vi "浊度电极校准.vi"() -> ()   [LabVIEW 2016, in "斯坦道多参数.lvlib"]
uses:
  <vilib>/Utility/miscctls.llb/LVPointTypeDef.ctl
  <vilib>/Utility/miscctls.llb/LVPositionTypeDef.ctl
  <vilib>/Analysis/NI_AALBase.lvlib
panel:
  out "第三点校准值":dbl
  out "标液3":dbl
  out "第二点校准值":dbl
  out "第一点校准值":dbl
  in  "校准停止":bool
  in  "校准启动":bool
  in  "校准模式":enum16{"两点校准", "单点校准", "三点校准"}(ring)
  out "最小值":sgl format="%#.2f"
  out "最大值":sgl format="%#.2f"
  out "波形图表":sgl(graph) caption="历史曲线"
  out "mean":dbl caption="均值" format="%#.2f"
  out "standard deviation":dbl caption="标准差" format="%#.2f"
  out "变异系数":dbl format="%#.6f"
  out "测量值":dbl
  out "提示":string
  out "标液2":dbl
  out "标液1":dbl
  out "原始读取值":dbl caption="信号值"
  out "偏移值补偿":dbl
  out "电极斜率":dbl
  out "电极零点":dbl
  # "浊度电极设定"
  # "NTU"
  # "%"
  # "NTU"
  # "NTU"
  # "NTU"
  # "请选择校准模式:"
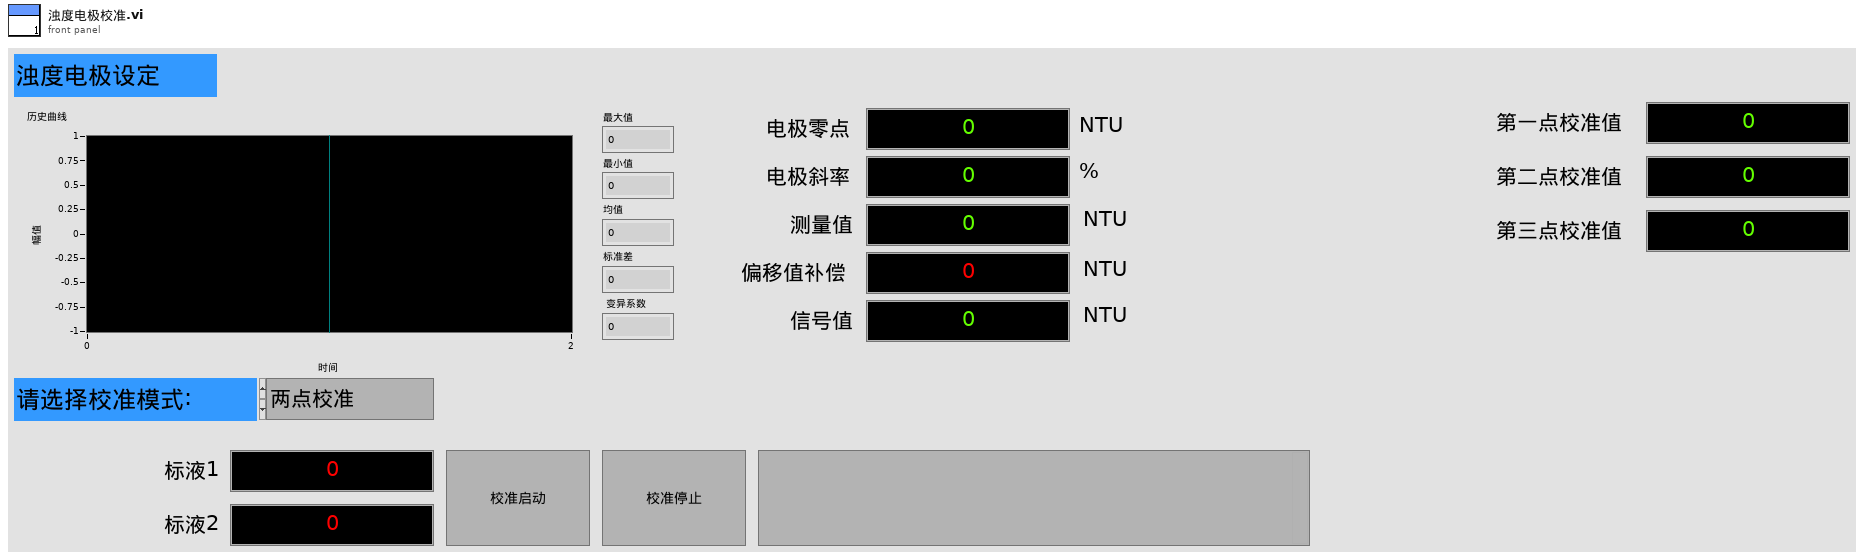
[diagram p1: front panel]
types:
  T1 = typedef "LVPointTypeDef.ctl" = cluster{"Horizontal":i16, "Vertical":i16}
  T2 = typedef "斯坦道多参数.lvlib/校准步骤.ctl" = enum16{"待机", "放置第一点标液", "第一点校准启动", "第一点校准写入", "第一点校准失败", "放置第二点标液", "第二点校准启动", "第二点校准写入", "第二点校准失败", "放置第三点标液", "第三点校准启动", "第三点校准写入", "第三点校准失败", "校准结果写入", "校准结束"}
  T3 = cluster{"电极状态标志":u16, "电极型号标志":u16, "浊度测量值":sgl, "温度测量值":sgl, "浊度信号值":sgl, "浊度偏移修正值":sgl, "温度偏移修正值":sgl, "手动温度补偿值":sgl, "浊度电极零点":sgl, "浊度电极斜率":sgl, "第1点标准值记录":sgl, "第1点信号值记录":sgl, "第1点温度值记录":sgl, "第2点标准值记录":sgl, "第2点信号值记录":sgl, "第2点温度值记录":sgl, "命令滤波设定":u16, "温度模式":enum16{"ATC", "MTC"}, "生产批次":u16, "电极序号":u16, "串口地址":u16, "串口波特率":enum16{"9600", "19200", "115200"}, "串口校验位":enum16{"NONE", "ODD", "EVEN"}, "串口停止位":enum16{"1bit", "2bit"}, "第一点标准值":sgl, "第二点标准值":sgl, "第三点标准值":sgl}
  T4 = typedef "LVPositionTypeDef.ctl" = cluster{"Left":i32, "Top":i32}
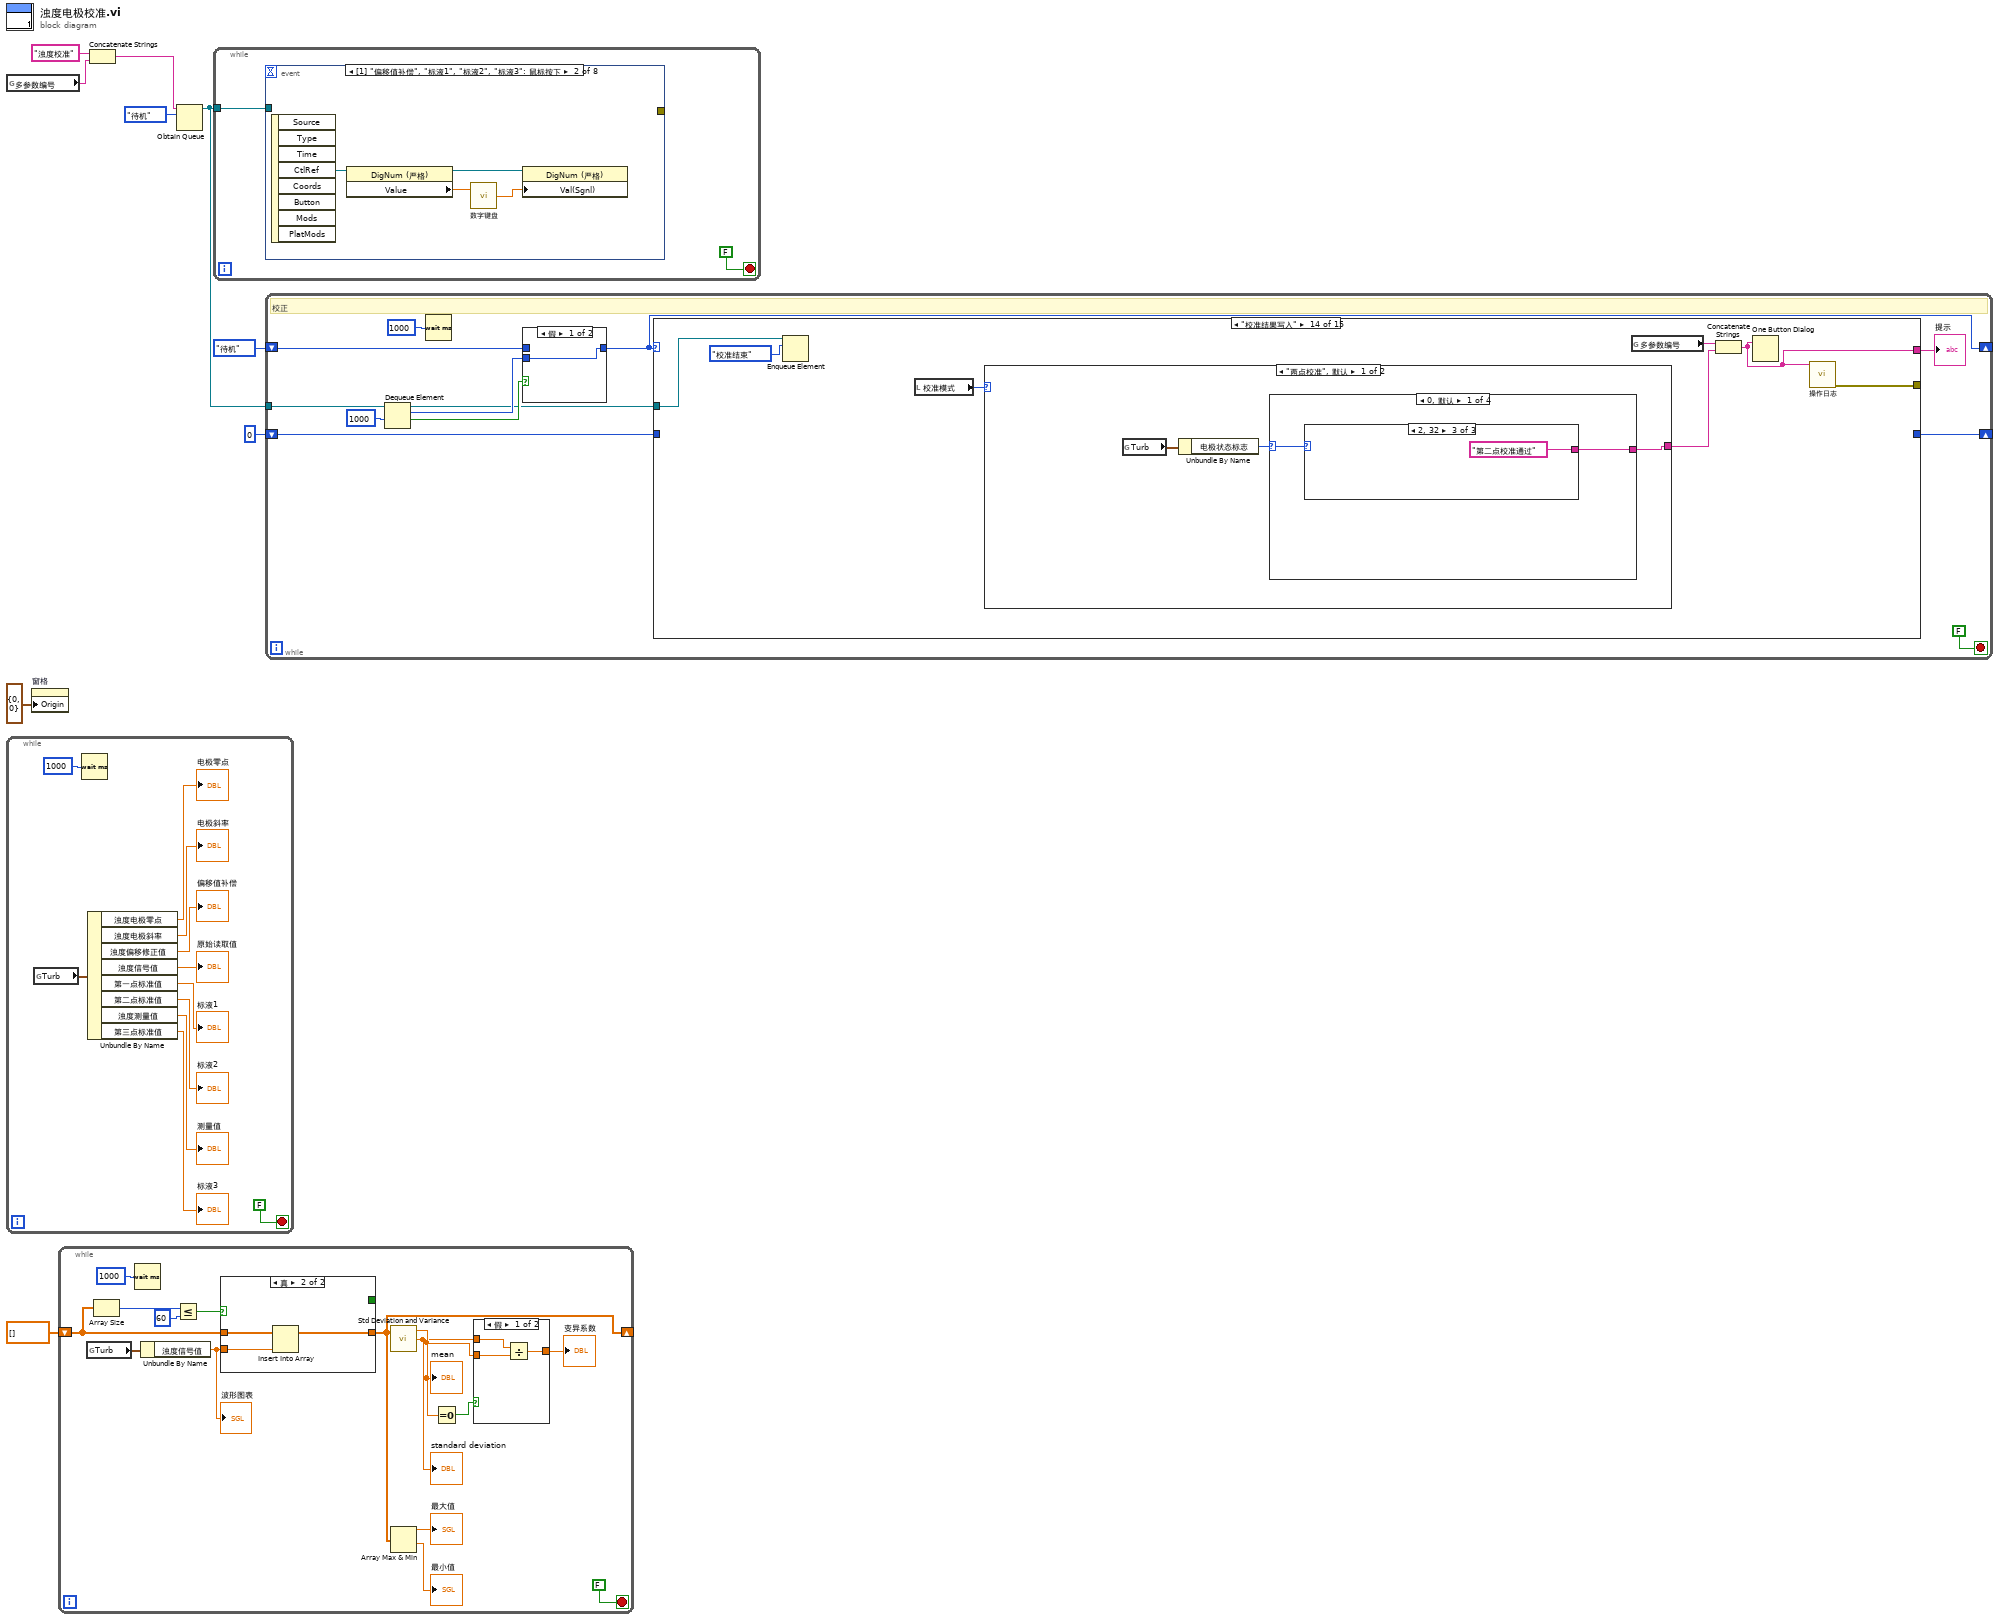
[diagram p0: block diagram]
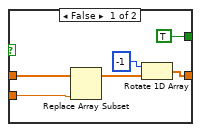
[diagram p3: hidden frame]
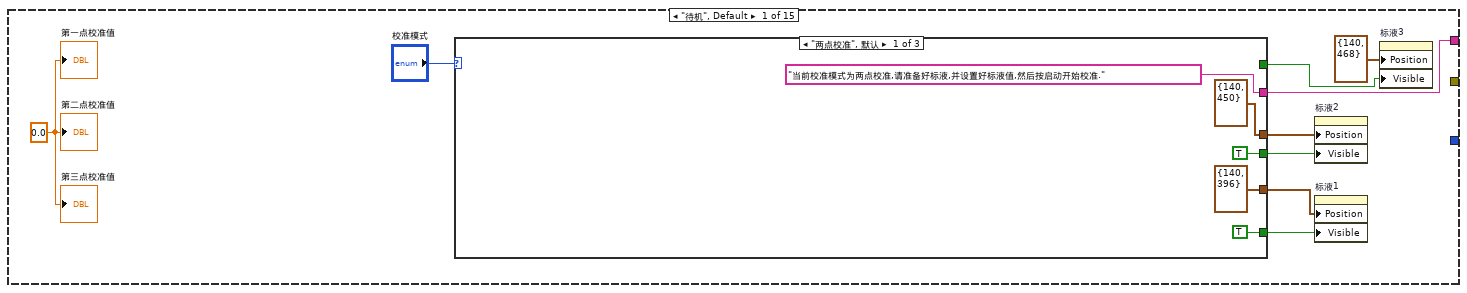
[diagram p5: hidden frame]
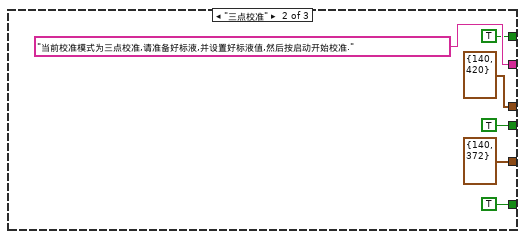
[diagram p6: hidden frame]
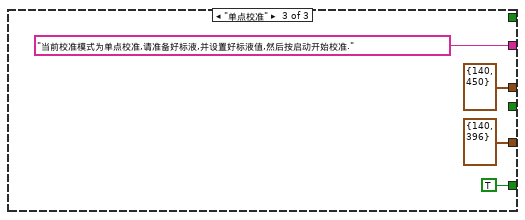
[diagram p7: hidden frame]
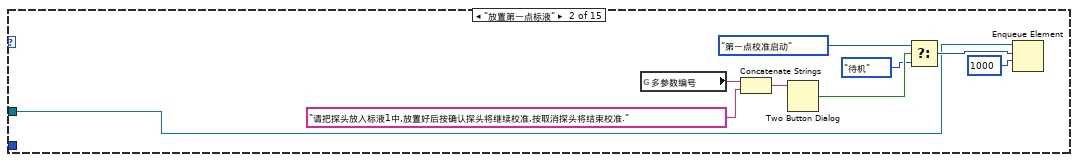
[diagram p8: hidden frame]
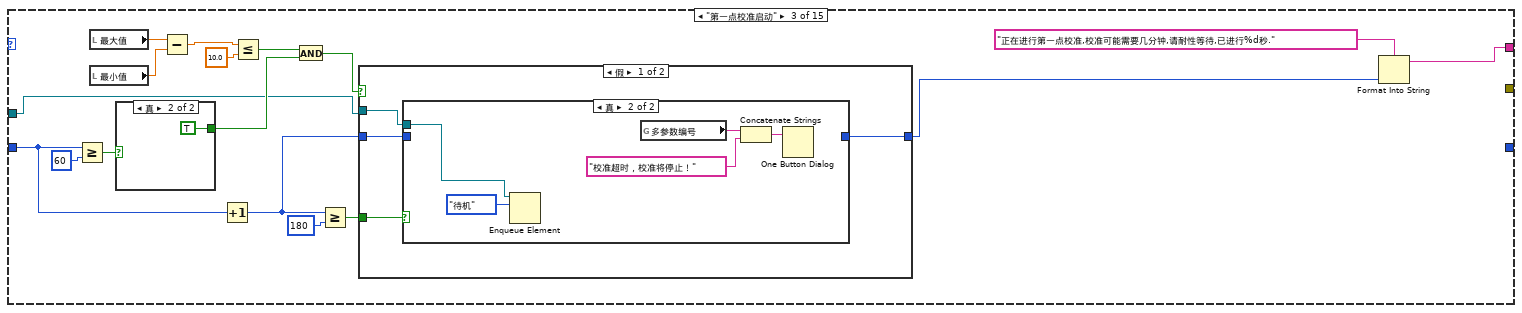
[diagram p9: hidden frame]
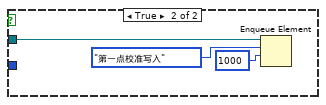
[diagram p11: hidden frame]
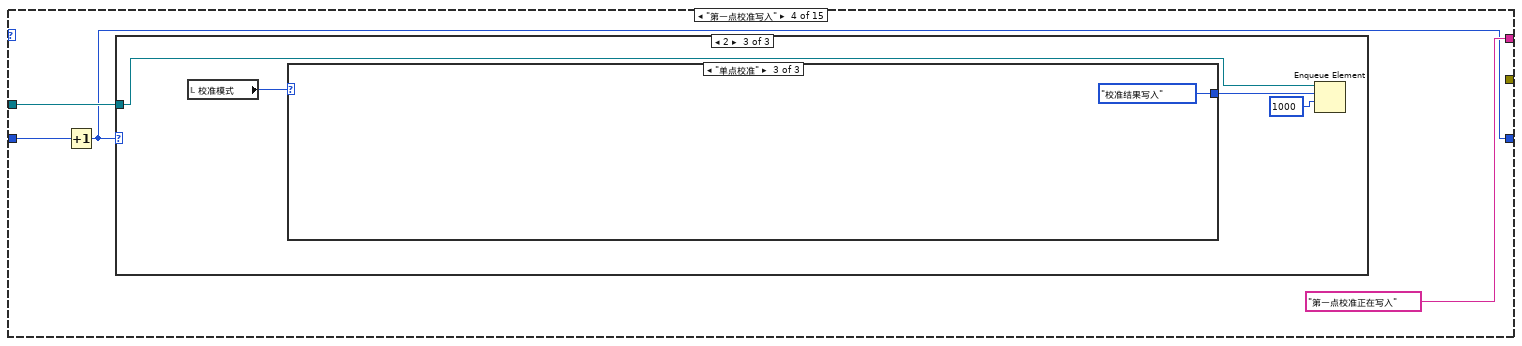
[diagram p13: hidden frame]
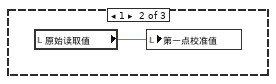
[diagram p15: hidden frame]
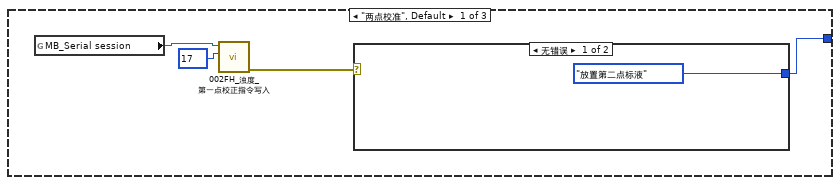
[diagram p16: hidden frame]
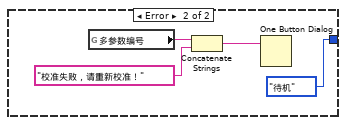
[diagram p17: hidden frame]
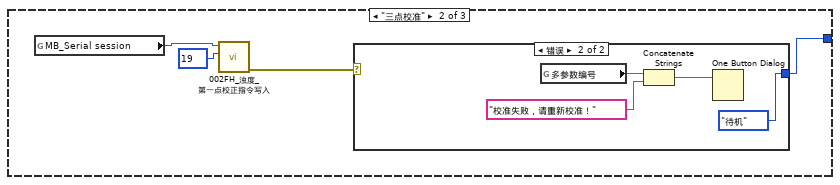
[diagram p18: hidden frame]
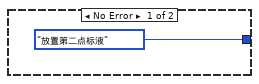
[diagram p19: hidden frame]
diagram:
  n1 = global read "多参数全局变量.vi" "多参数编号"() -> (w1:string)
  n2 = while {
    stop <- FALSE stop-if-true
    n3 = global read "国弘过程全局变量.vi" "Turb"() -> (w18:T3)
    n4 = Wait (ms)(milliseconds to wait=u32 1000 ("等待时间（毫秒）")) -> ()  [unwired: 1 out]
    n5 = Unbundle By Name(w18) -> ("浊度电极零点"=→"电极零点":sgl, "浊度电极斜率"=→"电极斜率":sgl, "浊度偏移修正值"=→"偏移值补偿":sgl, "浊度信号值"=→"原始读取值":sgl, "第一点标准值"=→"标液1":sgl, "第二点标准值"=→"标液2":sgl, "浊度测量值"=→"测量值":sgl, "第三点标准值"=→"标液3":sgl)
  }
  n6 = property on="窗格" class="Pane"("Origin"=T1 {"Horizontal"=0, "Vertical"=0} ("原点")) -> ()  [unwired: 2 in, 2 out]
  n7 = while {
    shift-right: [w24] -> _
    shift-left: sgl[] [] -> [w31]
    stop <- FALSE stop-if-true
    n8 = global read "国弘过程全局变量.vi" "Turb"() -> (w25:T3)
    n9 = Array Size(array=w31) -> (size(s)=w33:i32)
    n10 = Wait (ms)(milliseconds to wait=u32 1000 ("等待时间（毫秒）")) -> ()  [unwired: 1 out]
    n11 = Unbundle By Name(w25) -> ("浊度信号值"=w21:sgl)
    "波形图表" <- w21
    n12 = Less Or Equal?(x=w33, y=60) -> (x <= y?=w32:bool)
    n13 = case shown="真" w32 {
      tunnel: w31 -> [w44 w47]
      tunnel: w21 -> [w42 w46]
      tunnel: [w40 w45] -> w24
      tunnel: [TRUE _] -> _
      frame False {
        n14 = Replace Array Subset(array=w44, new element=w42) -> (w43:sgl[])  [unwired: 1 in]
        n15 = Rotate 1D Array(1:w43, 2:-1 ("n")) -> (0:w40:sgl[])
      }
      frame True {
        n16 = Insert Into Array(array=w47, new element=w46) -> (w45:sgl[])  [unwired: 1 in]
      }
    }
    n17 = call <vilib>:"Std Deviation and Variance.vi"("X"=w24) -> ("mean"=w29:dbl, "standard deviation"=w28:dbl)  [unwired: 1 in, 1 out]
    "mean" <- w29
    "standard deviation" <- w28
    n18 = Array Max & Min(array=w24) -> (max value=→"最大值":sgl, min value=→"最小值":sgl)  [unwired: 2 out]
    n19 = Equal To 0?(x=w29) -> (x = 0?=w30:bool)
    n20 = case shown="假" w30 {
      tunnel: w28 -> [w38 _]
      tunnel: [w37 _] -> w27
      tunnel: w29 -> [w36 _]
      frame False {
        n21 = Divide(x=w38, y=w36) -> (x/y=w37:dbl)
      }
      frame True {
      }
    }
    "变异系数" <- w27
  }
  n22 = Concatenate Strings("浊度校准" ("名称（未命名）"), w1) -> (w2:string)
  n23 = Obtain Queue(name (unnamed)=w2, element data type=校准步骤."待机" ("枚举")) -> (queue out=w4:refnum<queue>)  [unwired: 3 in, 2 out]
  n24 = while {
    tunnel: w4 -> [w48]
    stop <- FALSE stop-if-true
    n25 = event shown="[1] \"偏移值补偿\", \"标液1\", \"标液2\", \"标液3\": 鼠标按下" {
      selector: _ -> [_ _ _ _ _ _ _ _]
      dyn-events: _ -> [_ _ _ _ _ _ _ _]
      timeout: _ -> [_ _ _ _ _ _ _ _]
      tunnel: [_ _ w55 w58 w62 w65 _ _] -> _
      tunnel: w48 -> [_ _ _ _ _ _ w66 w68]
      event Timeout {
        n26 = event-data() -> ()  [unwired: 1 in, 3 out]
      }
      event "偏移值补偿", "标液1", "标液2", "标液3": Mouse Down {
        n27 = event-data() -> ("CtlRef"=w50:refnum<vi>)  [unwired: 1 in, 7 out]
        n28 = property class="DigNum (严格)"(reference=w50) -> (reference out=w51:refnum<vi>, "Value"=w52:dbl)  [unwired: 1 in, 1 out]
        n29 = call "数字键盘.vi"("OldNumber"=w52) -> ("NewNumber"=w53:dbl)  [unwired: 1 in]
        n30 = property class="DigNum (严格)"(reference=w51, "Val(Sgnl)"=w53) -> ()  [unwired: 1 in, 2 out]
      }
      event "偏移值补偿": Value Change {
        n31 = event-data() -> ("NewVal"=w56:dbl)  [unwired: 1 in, 5 out]
        n32 = global read "多参数全局变量.vi" "MB_Serial session"() -> (w54:refnum<class "MB_Master_Serial.lvclass">)
        n33 = call "000CH_浊度_浊度偏移修正值写入.vi"("数值"=w56, "MB_Serial session in"=w54) -> ("error out"=w55:errorcluster)  [unwired: 8 in, 1 out]
      }
      event "标液1": Value Change {
        n34 = event-data() -> ("NewVal"=w59:dbl)  [unwired: 1 in, 5 out]
        n35 = global read "多参数全局变量.vi" "MB_Serial session"() -> (w57:refnum<class "MB_Master_Serial.lvclass">)
        n36 = call "0030H_浊度_第一点标准值写入.vi"("数值"=w59, "MB_Serial session in"=w57) -> ("error out"=w58:errorcluster)  [unwired: 8 in, 1 out]
      }
      event "标液2": Value Change {
        n37 = event-data() -> ("NewVal"=w61:dbl)  [unwired: 1 in, 5 out]
        n38 = global read "多参数全局变量.vi" "MB_Serial session"() -> (w60:refnum<class "MB_Master_Serial.lvclass">)
        n39 = call "0033H_浊度_第二点标准值写入.vi"("数值"=w61, "MB_Serial session in"=w60) -> ("error out"=w62:errorcluster)  [unwired: 8 in, 1 out]
      }
      event "标液3": Value Change {
        n40 = event-data() -> ("NewVal"=w64:dbl)  [unwired: 1 in, 5 out]
        n41 = global read "多参数全局变量.vi" "MB_Serial session"() -> (w63:refnum<class "MB_Master_Serial.lvclass">)
        n42 = call "0036H_浊度_第三点标准值写入.vi"("数值"=w64, "MB_Serial session in"=w63) -> ("error out"=w65:errorcluster)  [unwired: 8 in, 1 out]
      }
      event "校准启动": Value Change {
        n43 = event-data() -> ()  [unwired: 1 in, 6 out]
        n44 = Enqueue Element(queue=w66, element=校准步骤."放置第一点标液" ("元素")) -> ()  [unwired: 2 in, 3 out]
      }
      event "校准停止": Value Change {
        n45 = event-data() -> ()  [unwired: 1 in, 6 out]
        n46 = Flush Queue(queue=w68) -> (queue out=w69:refnum<queue>)  [unwired: 1 in, 2 out]
        n47 = Enqueue Element(queue=w69, element=校准步骤."待机" ("元素"), timeout in ms (-1)=1000 ("超时毫秒(-1)")) -> ()  [unwired: 1 in, 3 out]
      }
    }
  }
  n48 = while "While循环" {
    shift-right: [w73] -> _
    shift-left: 校准步骤."待机" ("枚举") -> [w75]
    shift-right: [w72] -> _
    shift-left: 0 -> [w81]
    tunnel: w4 -> [w76]
    stop <- FALSE stop-if-true
    # "校正"
    n49 = Dequeue Element(queue=w76, timeout in ms (-1)=1000 ("超时毫秒(-1)")) -> (queue out=w74:refnum<queue>, element=w77:T2, timed out?=w78:bool)  [unwired: 1 in, 1 out]
    n50 = Wait (ms)(milliseconds to wait=u32 1000 ("等待时间（毫秒）")) -> ()  [unwired: 1 out]
    n51 = case shown="假" w78 {
      tunnel: w77 -> [w84 _]
      tunnel: [w84 w85] -> w73
      tunnel: w75 -> [_ w85]
      frame False {
      }
      frame True {
      }
    }
    n52 = case shown="\"校准结果写入\"" w73 {
      tunnel: [w93 _ w119 "第一点校准正在写入" ("提示") _ _ w189 "第二点校准正在写入" ("提示") "第二点校准失败" ("提示") _ "第三点校准正在写入" ("提示") w273 "第三点校准失败" ("提示") w304 w342] -> w80
      tunnel: w81 -> [_ _ w121 w152 _ _ w190 w220 _ _ w257 w274 _ _ _]
      tunnel: [_ _ _ w150 _ _ w188 w218 _ _ w255 w272 _ _ _] -> w72
      tunnel: w74 -> [_ w112 w122 w151 _ w180 w191 w219 _ w248 w256 w275 _ w308 _]
      tunnel: [_ _ _ _ _ _ _ _ _ _ _ _ _ w303 _] -> _
      frame "待机", Default {
        w86 = 0.0 ("第一点校准值")
        n53 = case shown="\"两点校准\", 默认" "校准模式" {
          tunnel: ["当前校准模式为两点校准,请准备好标液,并设置好标液值,然后按启动开始校准." ("提示") "当前校准模式为三点校准,请准备好标液,并设置好标液值,然后按启动开始校准." ("提示") "当前校准模式为单点校准,请准备好标液,并设置好标液值,然后按启动开始校准." ("提示")] -> w93
          tunnel: [TRUE ("可见") TRUE ("可见") _] -> w89
          tunnel: [T4 {"Left"=140, "Top"=396} ("位置") T4 {"Left"=140, "Top"=372} ("位置") T4 {"Left"=140, "Top"=396} ("位置")] -> w92
          tunnel: [T4 {"Left"=140, "Top"=450} ("位置 2") T4 {"Left"=140, "Top"=420} ("位置 2") T4 {"Left"=140, "Top"=450} ("位置 2")] -> w91
          tunnel: [_ TRUE ("可见") _] -> w88
          tunnel: [TRUE ("可见") TRUE ("可见") TRUE ("可见")] -> w87
          frame "两点校准", Default {
          }
          frame "三点校准" {
          }
          frame "单点校准" {
          }
        }
        n54 = property on="标液2" class="DigNum (严格)"("Position"=w91, "Visible"=w89) -> ()  [unwired: 2 in, 2 out]
        n55 = property on="标液1" class="DigNum (严格)"("Position"=w92, "Visible"=w87) -> ()  [unwired: 2 in, 2 out]
        n56 = property on="标液3" class="DigNum (严格)"("Position"=T4 {"Left"=140, "Top"=468} ("位置 3"), "Visible"=w88) -> ()  [unwired: 2 in, 2 out]
        "第一点校准值" <- w86
        "第二点校准值" <- w86
        "第三点校准值" <- w86
      }
      frame "放置第一点标液" {
        n57 = global read "多参数全局变量.vi" "多参数编号"() -> (w110:string)
        n58 = Concatenate Strings(w110, "请把探头放入标液1中,放置好后按确认探头将继续校准,按取消探头将结束校准." ("消息")) -> (w111:string)
        n59 = Two Button Dialog(message=w111) -> (T button?=w116:bool)  [unwired: 2 in]
        n60 = Select(t=校准步骤."第一点校准启动" ("元素"), s=w116, f=校准步骤."待机" ("元素")) -> (s? t:f=w113:T2)
        n61 = Enqueue Element(queue=w112, element=w113, timeout in ms (-1)=1000 ("超时毫秒(-1)")) -> ()  [unwired: 1 in, 3 out]
      }
      frame "第一点校准启动" {
        n62 = Greater Or Equal?(x=w121, y=60) -> (x >= y?=w128:bool)
        n63 = local read "最大值"() -> (w131:sgl)
        n64 = local read "最小值"() -> (w130:sgl)
        n65 = case shown="真" w128 {
          tunnel: [_ TRUE] -> w129
          frame False {
          }
          frame True {
          }
        }
        n66 = Subtract(x=w131, y=w130) -> (x-y=w132:sgl)
        n67 = Increment(x=w121) -> (x+1=w135:i32)
        n68 = Less Or Equal?(x=w132, y=10.0) -> (x <= y?=w125:bool)
        n69 = And(x=w125, y=w129) -> (x .and. y?=w133:bool)
        n70 = Greater Or Equal?(x=w135, y=180) -> (x >= y?=w134:bool)
        n71 = case shown="假" w133 {
          tunnel: w122 -> [w138 w148]
          tunnel: w134 -> [w139 _]
          tunnel: w135 -> [w137 _]
          tunnel: [w136 _] -> w120
          frame False {
            n72 = case shown="真" w139 {
              tunnel: w138 -> [_ w145]
              tunnel: w137 -> [w140 _]
              tunnel: [w140 _] -> w136
              frame False {
              }
              frame True {
                n73 = Enqueue Element(queue=w145, element=校准步骤."待机" ("元素")) -> ()  [unwired: 2 in, 3 out]
                n74 = global read "多参数全局变量.vi" "多参数编号"() -> (w141:string)
                n75 = Concatenate Strings(w141, "校准超时，校准将停止！" ("消息")) -> (w142:string)
                n76 = One Button Dialog(message=w142) -> ()  [unwired: 1 in, 1 out]
              }
            }
          }
          frame True {
            n77 = Enqueue Element(queue=w148, element=校准步骤."第一点校准写入" ("元素"), timeout in ms (-1)=1000 ("超时毫秒(-1)")) -> ()  [unwired: 1 in, 3 out]
          }
        }
        n78 = Format Into String(format string="正在进行第一点校准,校准可能需要几分钟,请耐性等待,已进行%d秒." ("格式字符串"), w120) -> (resulting string=w119:string)  [unwired: 2 in, 1 out]
      }
      frame "第一点校准写入" {
        n79 = Increment(x=w152) -> (x+1=w150:i32)
        n80 = case shown="2" w150 {
          tunnel: w151 -> [_ _ w158]
          frame 0, Default {
          }
          frame 1 {
            n81 = local read "原始读取值"() -> (w154:dbl)
            n82 = local write "第一点校准值"(w154) -> ()
          }
          frame 2 {
            n83 = local read "校准模式"() -> (w157:enum16{"两点校准", "单点校准", "三点校准"})
            n84 = case shown="\"单点校准\"" w157 {
              tunnel: [w159 w168 校准步骤."校准结果写入" ("元素")] -> w156
              frame "两点校准", Default {
                n85 = global read "多参数全局变量.vi" "MB_Serial session"() -> (w162:refnum<class "MB_Master_Serial.lvclass">)
                n86 = call "002FH_浊度_第一点校正指令写入.vi"("数值"=u16 17, "MB_Serial session in"=w162) -> ("error out"=w160:errorcluster)  [unwired: 8 in, 1 out]
                n87 = case shown="无错误" w160 {
                  tunnel: [校准步骤."放置第二点标液" ("元素") 校准步骤."待机" ("元素")] -> w159
                  frame No Error {
                  }
                  frame Error {
                    n88 = global read "多参数全局变量.vi" "多参数编号"() -> (w164:string)
                    n89 = Concatenate Strings(w164, "校准失败，请重新校准！" ("消息")) -> (w165:string)
                    n90 = One Button Dialog(message=w165) -> ()  [unwired: 1 in, 1 out]
                  }
                }
              }
              frame "三点校准" {
                n91 = global read "多参数全局变量.vi" "MB_Serial session"() -> (w171:refnum<class "MB_Master_Serial.lvclass">)
                n92 = call "002FH_浊度_第一点校正指令写入.vi"("数值"=u16 19, "MB_Serial session in"=w171) -> ("error out"=w169:errorcluster)  [unwired: 8 in, 1 out]
                n93 = case shown="错误" w169 {
                  tunnel: [校准步骤."放置第二点标液" ("元素") 校准步骤."待机" ("元素")] -> w168
                  frame No Error {
                  }
                  frame Error {
                    n94 = global read "多参数全局变量.vi" "多参数编号"() -> (w173:string)
                    n95 = Concatenate Strings(w173, "校准失败，请重新校准！" ("消息")) -> (w174:string)
                    n96 = One Button Dialog(message=w174) -> ()  [unwired: 1 in, 1 out]
                  }
                }
              }
              frame "单点校准" {
              }
            }
            n97 = Enqueue Element(queue=w158, element=w156, timeout in ms (-1)=1000 ("超时毫秒(-1)")) -> ()  [unwired: 1 in, 3 out]
          }
        }
      }
      frame "第一点校准失败" {
      }
      frame "放置第二点标液" {
        n98 = global read "多参数全局变量.vi" "多参数编号"() -> (w178:string)
        n99 = Concatenate Strings(w178, "请把探头放入标液2中,放置好后按确认探头将继续校准,按取消探头将结束校准." ("消息")) -> (w179:string)
        n100 = Two Button Dialog(message=w179) -> (T button?=w184:bool)  [unwired: 2 in]
        n101 = Select(t=校准步骤."第二点校准启动" ("元素"), s=w184, f=校准步骤."待机" ("元素")) -> (s? t:f=w181:T2)
        n102 = Enqueue Element(queue=w180, element=w181, timeout in ms (-1)=1000 ("超时毫秒(-1)")) -> ()  [unwired: 1 in, 3 out]
      }
      frame "第二点校准启动" {
        n103 = Greater Or Equal?(x=w190, y=60) -> (x >= y?=w196:bool)
        n104 = local read "最大值"() -> (w199:sgl)
        n105 = local read "最小值"() -> (w198:sgl)
        n106 = case shown="真" w196 {
          tunnel: [_ TRUE] -> w197
          frame False {
          }
          frame True {
          }
        }
        n107 = Subtract(x=w199, y=w198) -> (x-y=w200:sgl)
        n108 = Increment(x=w190) -> (x+1=w203:i32)
        n109 = Less Or Equal?(x=w200, y=10.0) -> (x <= y?=w193:bool)
        n110 = And(x=w193, y=w197) -> (x .and. y?=w201:bool)
        n111 = Greater Or Equal?(x=w203, y=180) -> (x >= y?=w202:bool)
        n112 = case shown="假" w201 {
          tunnel: w191 -> [w206 w216]
          tunnel: w202 -> [w207 _]
          tunnel: w203 -> [w205 _]
          tunnel: [w204 _] -> w188
          frame False {
            n113 = case shown="真" w207 {
              tunnel: w206 -> [_ w213]
              tunnel: w205 -> [w208 _]
              tunnel: [w208 _] -> w204
              frame False {
              }
              frame True {
                n114 = Enqueue Element(queue=w213, element=校准步骤."放置第二点标液" ("元素")) -> ()  [unwired: 2 in, 3 out]
                n115 = global read "多参数全局变量.vi" "多参数编号"() -> (w209:string)
                n116 = Concatenate Strings(w209, "校准超时，校准将停止！" ("消息")) -> (w210:string)
                n117 = One Button Dialog(message=w210) -> ()  [unwired: 1 in, 1 out]
              }
            }
          }
          frame True {
            n118 = Enqueue Element(queue=w216, element=校准步骤."第二点校准写入" ("元素"), timeout in ms (-1)=1000 ("超时毫秒(-1)")) -> ()  [unwired: 1 in, 3 out]
          }
        }
        n119 = Format Into String(format string="正在进行第二点校准,校准可能需要几分钟,请耐性等待,已进行%d秒." ("格式字符串"), w188) -> (resulting string=w189:string)  [unwired: 2 in, 1 out]
      }
      frame "第二点校准写入" {
        n120 = Increment(x=w220) -> (x+1=w218:i32)
        n121 = case shown="2" w218 {
          tunnel: w219 -> [_ _ w226]
          frame 0, Default {
          }
          frame 1 {
            n122 = local read "原始读取值"() -> (w222:dbl)
            n123 = local write "第二点校准值"(w222) -> ()
          }
          frame 2 {
            n124 = local read "校准模式"() -> (w223:enum16{"两点校准", "单点校准", "三点校准"})
            n125 = case shown="\"两点校准\", 默认" w223 {
              tunnel: [w230 w239] -> w224
              frame "两点校准", Default {
                n126 = global read "多参数全局变量.vi" "MB_Serial session"() -> (w227:refnum<class "MB_Master_Serial.lvclass">)
                n127 = call "0032H_浊度_第二点校正指令写入.vi"("数值"=u16 33, "MB_Serial session in"=w227) -> ("error out"=w228:errorcluster)  [unwired: 8 in, 1 out]
                n128 = case shown="错误" w228 {
                  tunnel: [校准步骤."校准结果写入" ("元素") 校准步骤."放置第二点标液" ("元素")] -> w230
                  frame No Error {
                  }
                  frame Error {
                    n129 = global read "多参数全局变量.vi" "多参数编号"() -> (w232:string)
                    n130 = Concatenate Strings(w232, "校准失败，请重新校准！" ("消息")) -> (w233:string)
                    n131 = One Button Dialog(message=w233) -> ()  [unwired: 1 in, 1 out]
                  }
                }
              }
              frame "三点校准" {
                n132 = global read "多参数全局变量.vi" "MB_Serial session"() -> (w236:refnum<class "MB_Master_Serial.lvclass">)
                n133 = call "0032H_浊度_第二点校正指令写入.vi"("数值"=u16 35, "MB_Serial session in"=w236) -> ("error out"=w237:errorcluster)  [unwired: 8 in, 1 out]
                n134 = case shown="错误" w237 {
                  tunnel: [校准步骤."放置第三点标液" ("元素") 校准步骤."待机" ("元素")] -> w239
                  frame No Error {
                  }
                  frame Error {
                    n135 = global read "多参数全局变量.vi" "多参数编号"() -> (w241:string)
                    n136 = Concatenate Strings(w241, "校准失败，请重新校准！" ("消息")) -> (w242:string)
                    n137 = One Button Dialog(message=w242) -> ()  [unwired: 1 in, 1 out]
                  }
                }
              }
            }
            n138 = Enqueue Element(queue=w226, element=w224, timeout in ms (-1)=1000 ("超时毫秒(-1)")) -> ()  [unwired: 1 in, 3 out]
          }
        }
      }
      frame "第二点校准失败" {
      }
      frame "放置第三点标液" {
        n139 = global read "多参数全局变量.vi" "多参数编号"() -> (w246:string)
        n140 = Concatenate Strings(w246, "请把探头放入标液3中,放置好后按确认探头将继续校准,按取消探头将结束校准." ("消息")) -> (w247:string)
        n141 = Two Button Dialog(message=w247) -> (T button?=w252:bool)  [unwired: 2 in]
        n142 = Select(t=校准步骤."第三点校准启动" ("元素"), s=w252, f=校准步骤."待机" ("元素")) -> (s? t:f=w249:T2)
        n143 = Enqueue Element(queue=w248, element=w249, timeout in ms (-1)=1000 ("超时毫秒(-1)")) -> ()  [unwired: 1 in, 3 out]
      }
      frame "第三点校准写入" {
        n144 = Increment(x=w257) -> (x+1=w255:i32)
        n145 = case shown="2" w255 {
          tunnel: w256 -> [_ _ w265]
          frame 0, Default {
          }
          frame 1 {
            n146 = local read "原始读取值"() -> (w259:dbl)
            n147 = local write "第二点校准值"(w259) -> ()
          }
          frame 2 {
            n148 = global read "多参数全局变量.vi" "MB_Serial session"() -> (w260:refnum<class "MB_Master_Serial.lvclass">)
            n149 = call "0035H_浊度_第三点校正指令写入.vi"("数值"=u16 51, "MB_Serial session in"=w260) -> ("error out"=w261:errorcluster)  [unwired: 8 in, 1 out]
            n150 = case shown="无错误" w261 {
              tunnel: [校准步骤."校准结果写入" ("元素") 校准步骤."待机" ("元素")] -> w263
              frame No Error {
              }
              frame Error {
                n151 = global read "多参数全局变量.vi" "多参数编号"() -> (w267:string)
                n152 = Concatenate Strings(w267, "校准失败，请重新校准！" ("消息")) -> (w268:string)
                n153 = One Button Dialog(message=w268) -> ()  [unwired: 1 in, 1 out]
              }
            }
            n154 = Enqueue Element(queue=w265, element=w263, timeout in ms (-1)=1000 ("超时毫秒(-1)")) -> ()  [unwired: 1 in, 3 out]
          }
        }
      }
      frame "第三点校准启动" {
        n155 = Greater Or Equal?(x=w274, y=60) -> (x >= y?=w280:bool)
        n156 = local read "最大值"() -> (w283:sgl)
        n157 = local read "最小值"() -> (w282:sgl)
        n158 = case shown="真" w280 {
          tunnel: [_ TRUE] -> w281
          frame False {
          }
          frame True {
          }
        }
        n159 = Subtract(x=w283, y=w282) -> (x-y=w284:sgl)
        n160 = Increment(x=w274) -> (x+1=w287:i32)
        n161 = Less Or Equal?(x=w284, y=10.0) -> (x <= y?=w277:bool)
        n162 = And(x=w277, y=w281) -> (x .and. y?=w285:bool)
        n163 = Greater Or Equal?(x=w287, y=180) -> (x >= y?=w286:bool)
        n164 = case shown="假" w285 {
          tunnel: w275 -> [w290 w300]
          tunnel: w286 -> [w291 _]
          tunnel: w287 -> [w289 _]
          tunnel: [w288 _] -> w272
          frame False {
            n165 = case shown="真" w291 {
              tunnel: w290 -> [_ w297]
              tunnel: w289 -> [w292 _]
              tunnel: [w292 _] -> w288
              frame False {
              }
              frame True {
                n166 = Enqueue Element(queue=w297, element=校准步骤."待机" ("元素")) -> ()  [unwired: 2 in, 3 out]
                n167 = global read "多参数全局变量.vi" "多参数编号"() -> (w293:string)
                n168 = Concatenate Strings(w293, "校准超时，校准将停止！" ("消息")) -> (w294:string)
                n169 = One Button Dialog(message=w294) -> ()  [unwired: 1 in, 1 out]
              }
            }
          }
          frame True {
            n170 = Enqueue Element(queue=w300, element=校准步骤."第三点校准写入" ("元素"), timeout in ms (-1)=1000 ("超时毫秒(-1)")) -> ()  [unwired: 1 in, 3 out]
          }
        }
        n171 = Format Into String(format string="正在进行第三点校准,校准可能需要几分钟,请耐性等待,已进行%d秒." ("格式字符串"), w272) -> (resulting string=w273:string)  [unwired: 2 in, 1 out]
      }
      frame "第三点校准失败" {
      }
      frame "校准结果写入" {
        n172 = Enqueue Element(queue=w308, element=校准步骤."校准结束" ("元素")) -> ()  [unwired: 2 in, 3 out]
        n173 = local read "校准模式"() -> (w307:enum16{"两点校准", "单点校准", "三点校准"})
        n174 = case shown="\"两点校准\", 默认" w307 {
          tunnel: [w312 w336] -> w306
          frame "两点校准", Default {
            n175 = global read "国弘过程全局变量.vi" "Turb"() -> (w311:T3)
            n176 = Unbundle By Name(w311) -> ("电极状态标志"=w310:u16)
            n177 = case shown="0, 默认" w310 {
              selector: w310 -> [w314 _ _ w328]
              tunnel: [w313 w318 w323 w327] -> w312
              frame 0, Default {
                n178 = case shown="2, 32" w314 {
                  tunnel: ["校正未正常启动，请重新校正" "第一点校准通过" "第二点校准通过"] -> w313
                  frame 0, Default {
                  }
                  frame 1, 31 {
                  }
                  frame 2, 32 {
                  }
                }
              }
              frame 2 {
                n179 = local read "第一点校准值"() -> (w320:dbl)
                n180 = local read "第二点校准值"() -> (w321:dbl)
                n181 = Format Into String(format string="两点校准结果：\n第一点校准值：%f\n第二点校准值：%f" ("提示"), w320, w321) -> (resulting string=w318:string)  [unwired: 2 in, 1 out]
              }
              frame 33 {
                n182 = local read "第一点校准值"() -> (w325:dbl)
                n183 = local read "第二点校准值"() -> (w326:dbl)
                n184 = local read "第三点校准值"() -> (w322:dbl)
                n185 = Format Into String(format string="三点校准结果：\n第一点校准值：%f\n第二点校准值：%f\n第三点校准值：%f" ("提示"), w325, w326, w322) -> (resulting string=w323:string)  [unwired: 2 in, 1 out]
              }
              frame 3, 4 {
                n186 = case shown="3, 默认" w328 {
                  tunnel: ["校正失败，电极零点超出范围" "校正失败，电极斜率超出范围"] -> w327
                  frame 3, Default {
                  }
                  frame 4 {
                  }
                }
              }
            }
          }
          frame "单点校准" {
            n187 = local read "原始读取值"() -> (w335:dbl)
            n188 = local read "标液1"() -> (w334:dbl)
            n189 = global read "多参数全局变量.vi" "MB_Serial session"() -> (w333:refnum<class "MB_Master_Serial.lvclass">)
            n190 = Subtract(x=w334, y=w335) -> (x-y=w331:dbl)
            n191 = call "000CH_浊度_浊度偏移修正值写入.vi"("数值"=w331, "MB_Serial session in"=w333) -> ("error out"=w332:errorcluster)  [unwired: 8 in, 1 out]
            n192 = case shown="无错误" w332 {
              tunnel: [w337 "校准失败"] -> w336
              frame No Error {
                n193 = local read "第一点校准值"() -> (w339:dbl)
                n194 = Format Into String(format string="单点校准结果：\n校准值：%f" ("提示"), w339) -> (resulting string=w337:string)  [unwired: 2 in, 1 out]
              }
              frame Error {
                n195 = One Button Dialog(message="校准失败，请重新校准！" ("消息")) -> ()  [unwired: 1 in, 1 out]
              }
            }
          }
        }
        n196 = global read "多参数全局变量.vi" "多参数编号"() -> (w305:string)
        n197 = Concatenate Strings(w305, w306) -> (w304:string)
        n198 = One Button Dialog(message=w304) -> ()  [unwired: 1 in, 1 out]
        n199 = call "操作日志.vi"("日志信息"=w304) -> ("error out"=w303:errorcluster)  [unwired: 10 in]
      }
      frame "校准结束" {
        n200 = local read "提示"() -> (w342:string)
      }
    }
    "提示" <- w80
  }
